vi "Clock Synchronization Engine.vi"   [LabVIEW 2023]
doc: "This VI handles all timing stuff."
uses:
  <vilib>/Platform/TimedLoop/XDataNode/timing_clust.ctl
  <vilib>/Platform/TimedLoop/XDataNode/nitl_modes.ctl
  <vilib>/Platform/TimedLoop/XDataNode/wakeup.ctl
  Type Definitions/System Time.ctl
  Type Definitions/Payload Class.ctl
  Type Definitions/Enum - System State.ctl
  <vilib>/Utility/error.llb/Error Cluster From Error Code.vi
  <vilib>/rvi/errors/niLvFpgaAdjustHostInterfaceError.vi
  <vilib>/platform/TimedLoop/XDataNode/XDataNode.xnode
  <vilib>/rvi/interface/nirviReadWriteControl/nirviReadWriteControl.xnode
  <vilib>/Platform/TimedLoop/XDataNode/XDNodeRunTimeDep.lvlib
  <vilib>/rvi/interface/Simulation/niFpgaSimulationCallBeginRW.vi
  NiFpgaLv.dll
types:
  T1 = typedef "System Resources.ctl" = cluster{"System Session":refnum<k21>, "System Resource":refnum<k20>, "FPGA VI Reference":refnum<k20>}
  T2 = typedef "XDNodeRunTimeDep.lvlib/timing_clust.ctl" = cluster{"Expected End [f-1]":u64, "Actual End [f-1]":u64, "Finished Late? [f-1]":bool, "Expected End [i-1]":u64, "Actual End [i-1]":u64, "Finished Late? [i-1]":bool, "Expected Start [i]":u64, "Actual Start [i]":u64, "Expected Start [f]":u64, "Actual Start [f]":u64, "Source Name":string, "Structure Name":string, "Period":i64, "Deadline":i64, "Offset":i64, "Start":i64, "Priority":i32, "Timeout":i32, "Mode":T3, "Wakeup Reason":T4, "Error":errorcluster, "Source Type":string, "Secondary Source Type":string, "Global End Time":u64, "Global Start Time":u64, "Frame Duration":u64, "Iteration Duration":u64, "Assigned CPU":i32, "I/O Scan Engine Mode":u32}
  T3 = typedef "XDNodeRunTimeDep.lvlib/nitl_modes.ctl" = enum32{"No Change", "Process missed periods, maintain original phase", "Discard missed periods, maintain original phase", "Process missed periods, ignore original phase", "Discard missed periods, ignore original phase"}
  T4 = typedef "XDNodeRunTimeDep.lvlib/wakeup.ctl" = enum32{"Normal", "Aborted", "Asynchronous wakeup", "Timing source error", "Timed loop error", "Timeout"}
  T5 = typedef "Enum - System State.ctl" = enum16{"System Time", "Telemetry TCP State", "Writeable Drive State", "Command TCP State", "Network Adapter State", "Discovery Engine State", "Disk State"}
  T6 = typedef "Payload Class.ctl" = enum16{"System State", "Parameters", "Metadata", "Software Monitor", "Data", "Commands"}
  T7 = typedef "System Time.ctl" = cluster{"System Clock":timestamp, "GPS Clock":timestamp, "Nanosecond Counter":i64, "GPS Status":enum8{"Initializing", "Normal", "Unable to get fix"}, "GPS Antenna Status":enum8{"Unknown", "Normal", "Absent", "Overcurrent"}, "GPS Satelites Available":u8, "GPS Time (ns)":u64, "GPS UTC Offset":i8, "GPS Time Offset":i32, "UTC Offset Valid":bool, "GPS Time Lock":bool}
  T8 = enum8{"Initializing", "Normal", "Unable to get fix"}
  T9 = enum8{"Unknown", "Normal", "Absent", "Overcurrent"}
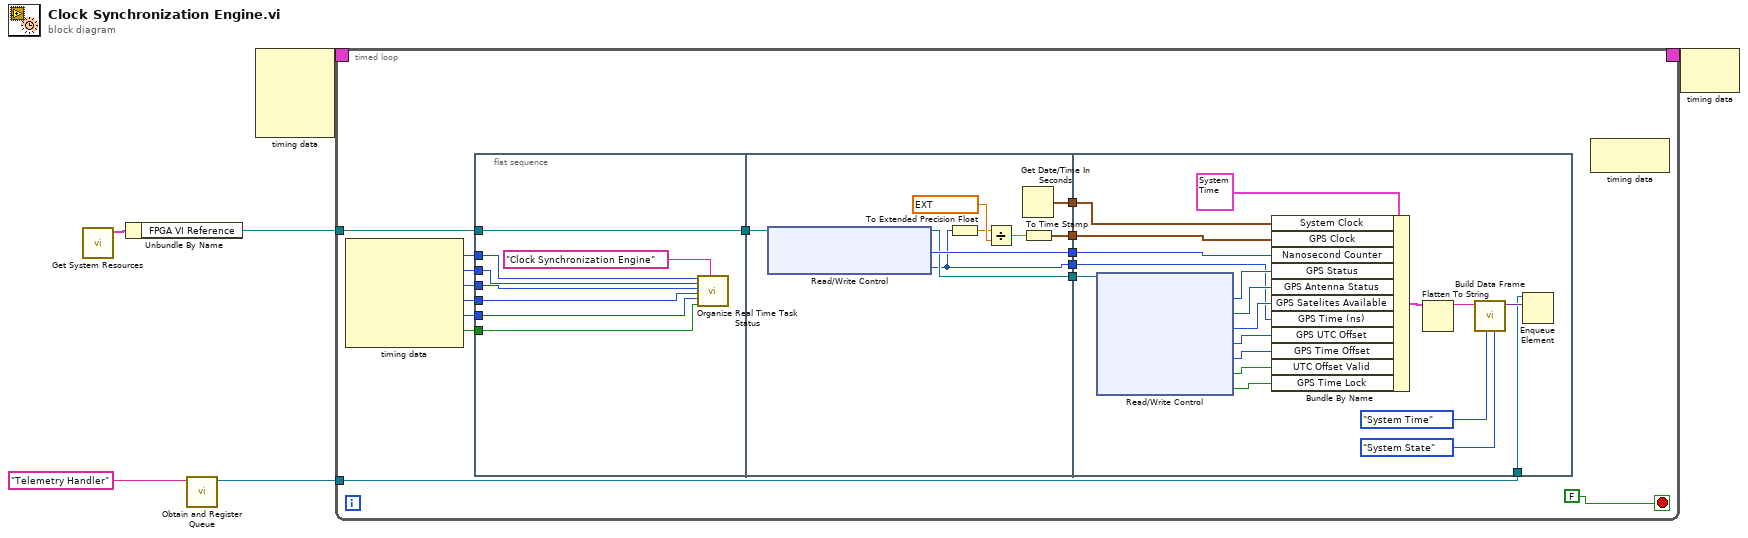
[diagram p0: block diagram]
diagram:
  n1 = call "Get System Resources.vi"() -> ("System Resources"=w2:T1)  [unwired: 10 in, 1 out]
  n2 = Unbundle By Name(w2) -> ("FPGA VI Reference"=w1:refnum<k20>)
  n3 = call "Obtain and Register Queue.vi"("Queue Name (unnamed)"="Telemetry Handler" ("name (unnamed)")) -> ("Queue Reference"=w6:refnum<queue>)  [unwired: 9 in, 1 out]
  n4 = node-c288() -> (w4:T2)  [unwired: 4 in]
  n5 = timed-loop {
    tunnel: w6 -> [w10]
    timing: w4 -> [_]
    timing-out: [_] -> w3
    tunnel: w1 -> [w20]
    stop <- FALSE stop-if-true
    n6 = node-c288() -> (w18:i32, w17:i32, w16:i64, w15:i64, w14:i64, w13:bool)  [unwired: 1 in]
    n7 = flat-sequence {
      tunnel: w20 -> [w29]
      tunnel: [w29] -> w19
      tunnel: w18 -> [w27]
      tunnel: w17 -> [w26]
      tunnel: w16 -> [w25]
      tunnel: w15 -> [w24]
      tunnel: w14 -> [w23]
      tunnel: w13 -> [w22]
      tunnel: w19 -> [w36]
      tunnel: [w38] -> w12
      tunnel: [w37] -> w11
      tunnel: [w35] -> w9
      tunnel: [w33] -> w8
      tunnel: [w30] -> w7
      tunnel: w12 -> [w50]
      tunnel: w11 -> [w49]
      tunnel: w10 -> [w53]
      tunnel: w9 -> [w52]
      tunnel: w8 -> [w44]
      tunnel: w7 -> [w39]
      frame #0 {
        n8 = call "Organize Real Time Task Status.vi"("Priority"=w27, "Processor"=w26, "Offset"=w25, "Iteration Duration"=w24, "Period"=w23, "Finished Late? [i-1]"=w22, "Task Name"="Clock Synchronization Engine") -> ()  [unwired: 12 in, 1 out]
      }
      frame #1 {
        n9 = xnode "Read/Write Control"("FPGA VI Reference In"=w36) -> ("FPGA VI Reference Out"=w35:refnum<k20>, "FPGA Nanosecond Counter"=w37:i64, "GPS Time (ns)"=w33:u64)  [unwired: 1 in, 1 out]
        n10 = To Extended Precision Float(1:w33) -> (0:w32:ext)
        n11 = Divide(x=w32, y=ext 1000000000.0) -> (x/y=w31:ext)
        n12 = Get Date/Time In Seconds() -> (seconds since 1Jan1904=w38:timestamp)
        n13 = To Time Stamp(1:w31) -> (0:w30:timestamp)
      }
      frame #2 {
        n14 = xnode "Read/Write Control"("FPGA VI Reference In"=w52) -> ("GPS Status"=w48:T8, "GPS Antenna Status"=w47:T9, "GPS Satelites Available"=w46:u8, "GPS UTC Offset"=w40:i8, "GPS Time Offset"=w45:i32, "GPS UTC Offset Valid"=w42:bool, "GPS Time Lock"=w41:bool)  [unwired: 1 in, 2 out]
        n15 = Bundle By Name(cluster=T7 {"System Clock"=timestamp(0 s since 1904-01-01), "GPS Clock"=timestamp(0 s since 1904-01-01), "Nanosecond Counter"=0, "GPS Status"=enum."Initializing", "GPS Antenna Status"=enum."Unknown", "GPS Satelites Available"=0, "GPS Time (ns)"=0, "GPS UTC Offset"=0, "GPS Time Offset"=0, "UTC Offset Valid"=FALSE, "GPS Time Lock"=FALSE}, "System Clock"=w50, "GPS Clock"=w39, "Nanosecond Counter"=w49, "GPS Status"=w48, "GPS Antenna Status"=w47, "GPS Satelites Available"=w46, "GPS Time (ns)"=w44, "GPS UTC Offset"=w40, "GPS Time Offset"=w45, "UTC Offset Valid"=w42, "GPS Time Lock"=w41) -> (w43:T7)
        n16 = Flatten To String(anything=w43) -> (data string=w54:string)  [unwired: 3 in, 2 out]
        n17 = call "Build Data Frame.vi"("Payload Class (Data)"=Payload_Class."System State", "Payload ID (0)"=Enum_-_System_State."System Time", "Payload (Empty String)"=w54) -> ("Frame"=w57:variant)  [unwired: 7 in, 1 out]
        n18 = Enqueue Element(queue=w53, element=w57) -> ()  [unwired: 2 in, 3 out]
      }
    }
    n19 = node-c288() -> ()  [unwired: 1 in, 1 out]
  }
  n20 = node-c288(w3) -> ()  [unwired: 1 out]
